vi "cDAQ - UI - Main.vi"() -> ()   [LabVIEW 2011]
uses:
  Controls/Init-Run-End States.ctl
  <vilib>/Utility/miscctls.llb/LVPointTypeDef.ctl
  SubVIs/Controls/TransparencyEffectOperations.ctl
panel:
  in  "Auto Mode":bool
  in  "stop":bool
  out "Picture 2":picture
  out "error out":errorcluster
  out "Picture":picture
  out "Default":picture
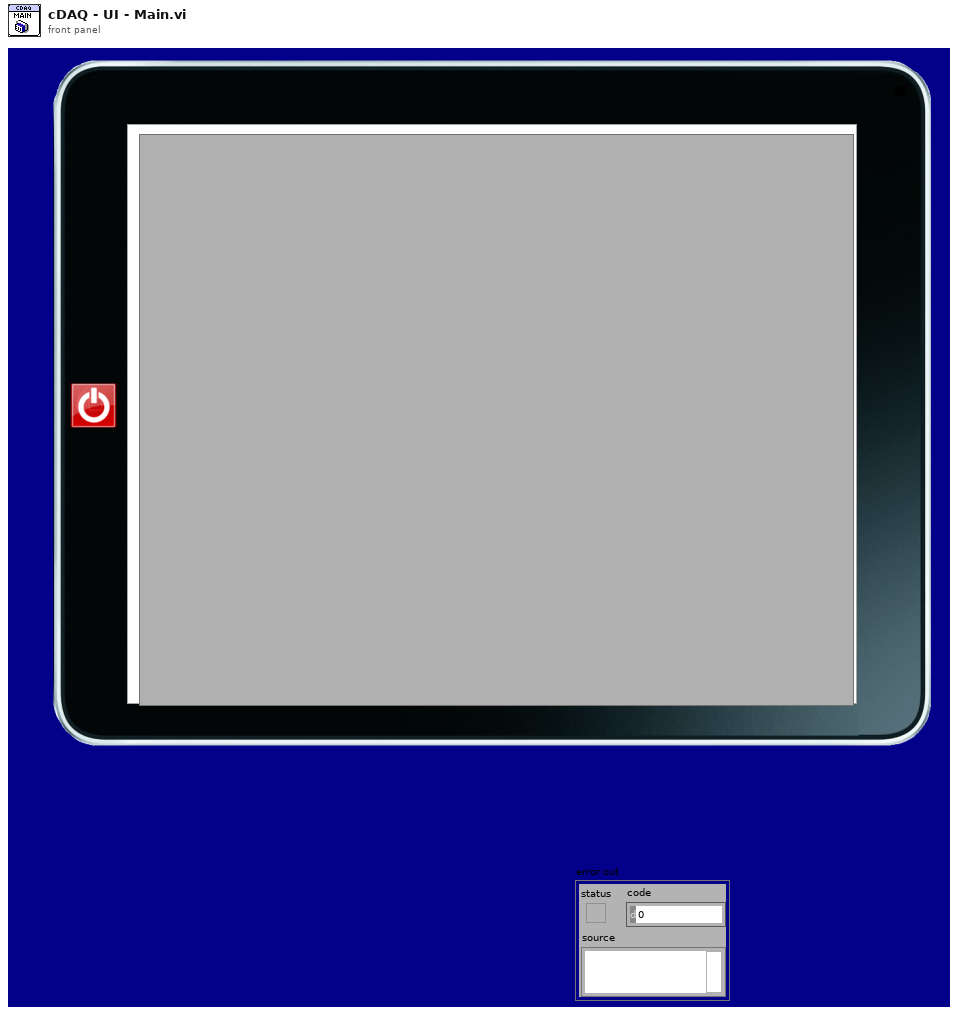
[diagram p1: front panel]
types:
  T1 = typedef "Init-Run-End States.ctl" = enum16{"INIT", "RUN", "END"}
  T2 = typedef "TransparencyEffectOperations.ctl" = enum16{"Show", "Hide 80%", "Hide All"}
  T3 = typedef "LVPointTypeDef.ctl" = cluster{"Horizontal":i16, "Vertical":i16}
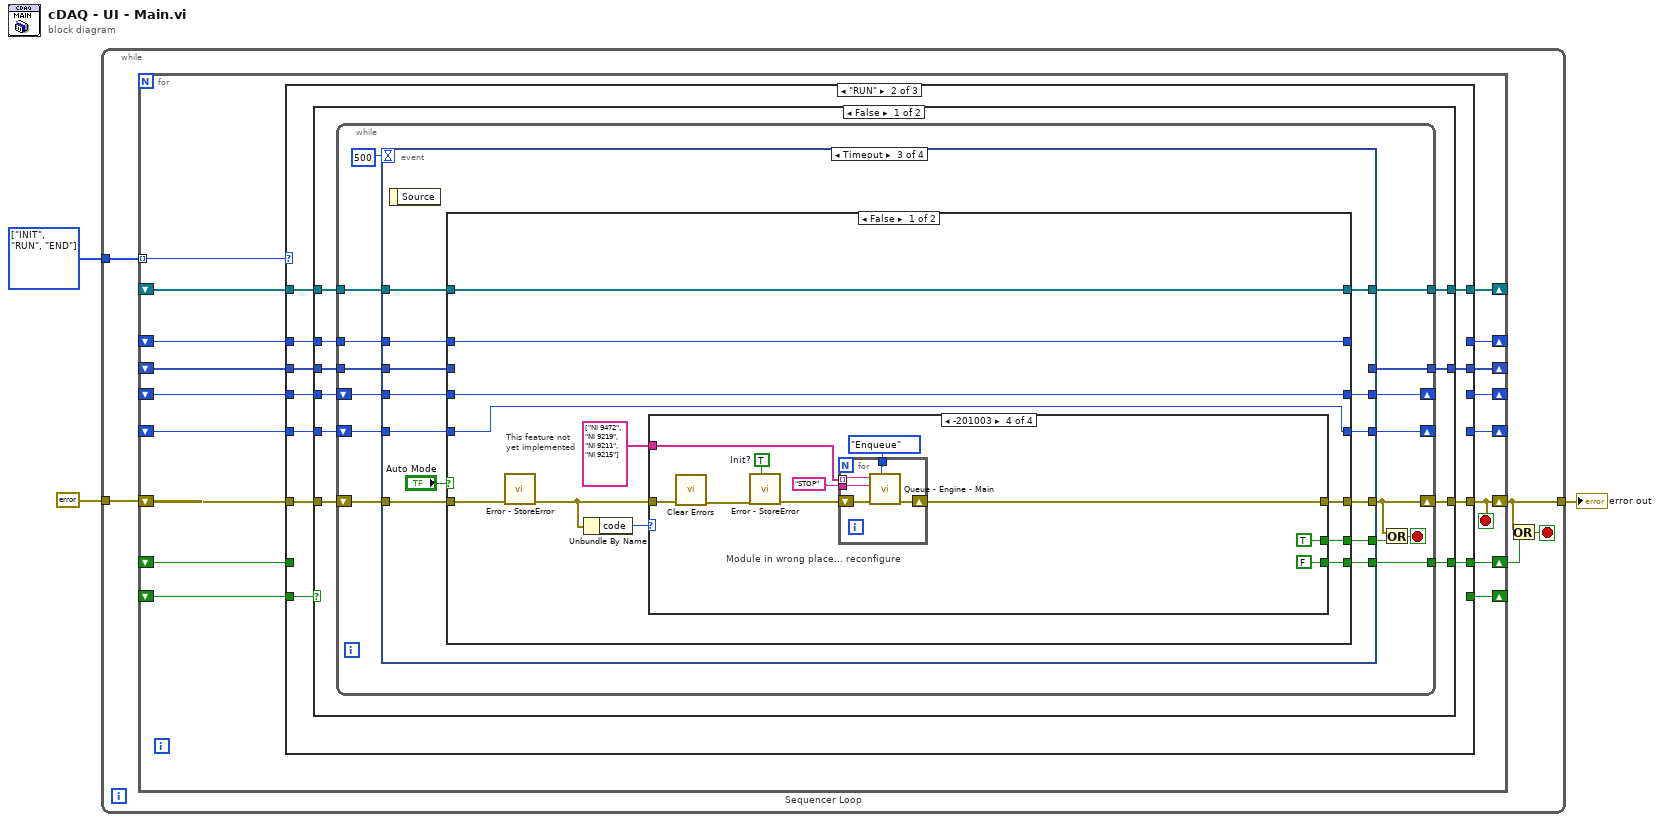
[diagram p0: block diagram]
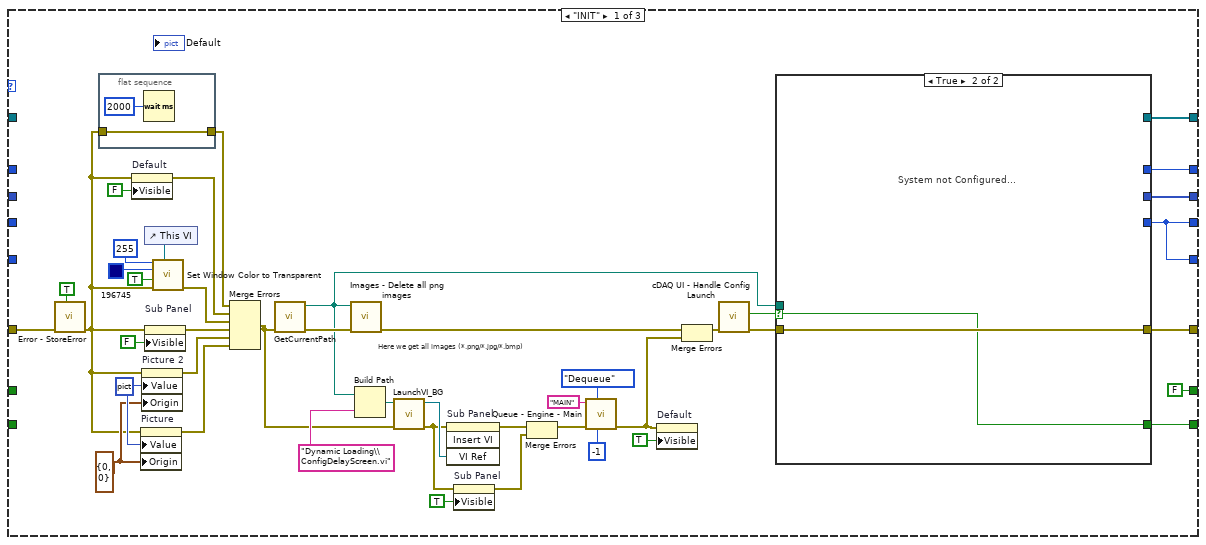
[diagram p2: hidden frame]
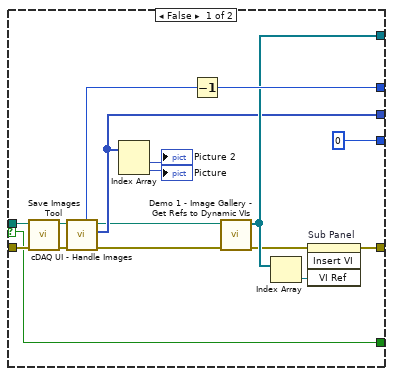
[diagram p3: hidden frame]
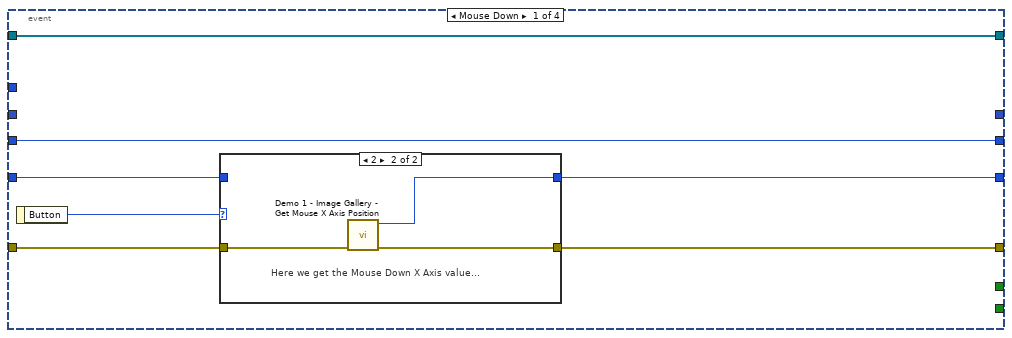
[diagram p4: hidden frame]
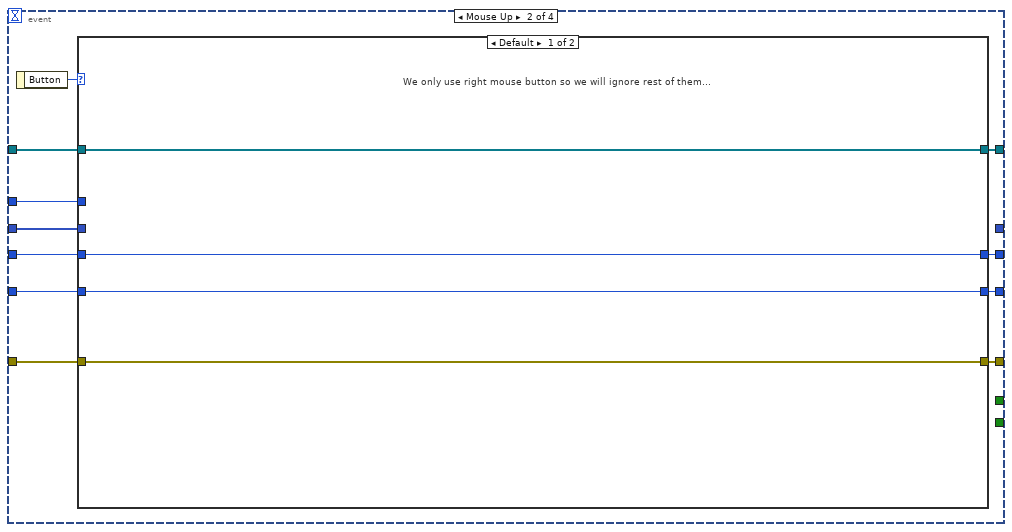
[diagram p6: hidden frame]
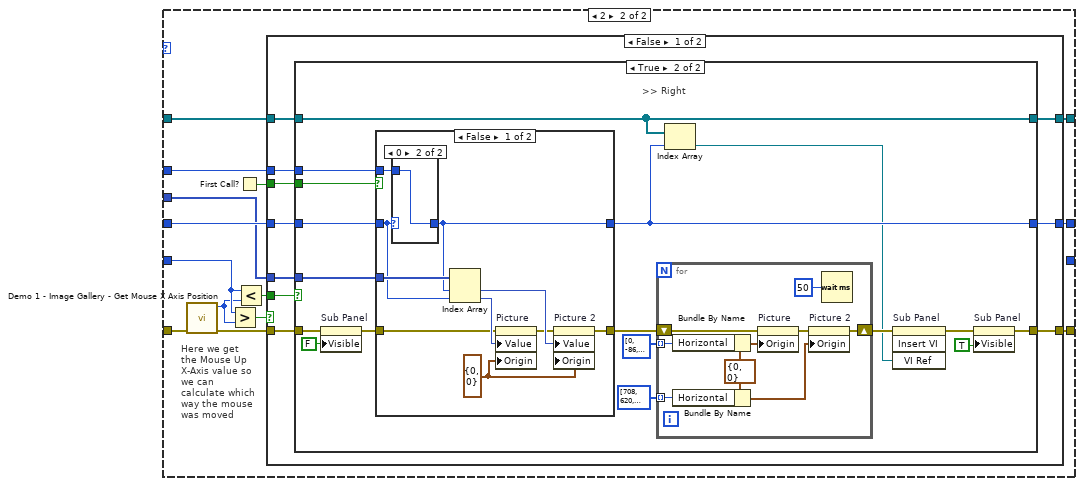
[diagram p7: hidden frame]
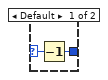
[diagram p9: hidden frame]
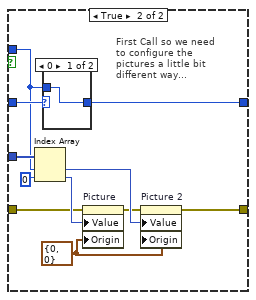
[diagram p10: hidden frame]
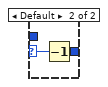
[diagram p11: hidden frame]
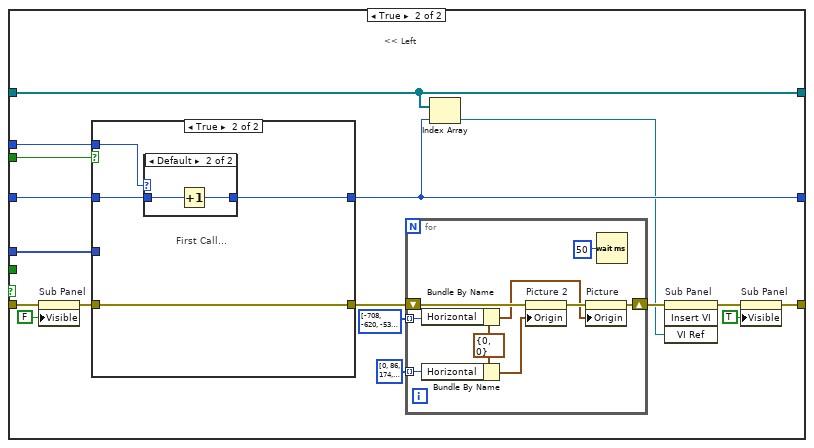
[diagram p12: hidden frame]
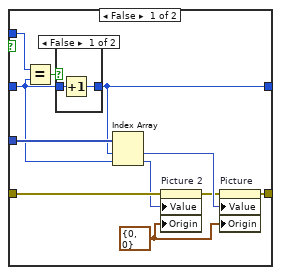
[diagram p13: hidden frame]
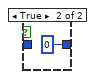
[diagram p14: hidden frame]
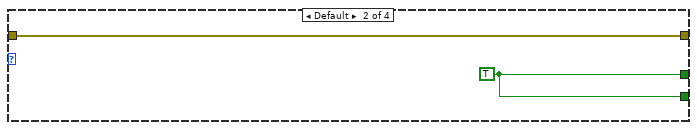
[diagram p17: hidden frame]
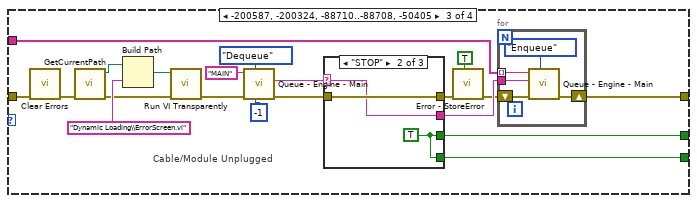
[diagram p18: hidden frame]
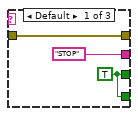
[diagram p19: hidden frame]
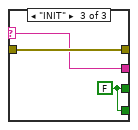
[diagram p20: hidden frame]
diagram:
  w3 = T1[] [enum."INIT", enum."RUN", enum."END"] items=["INIT", "RUN", "END"]
  n1 = while {
    tunnel: w3 -> [w8]
    tunnel: errorcluster {"status"=FALSE, "code"=0, "source"=""} ("error in (no error)") -> [w7]
    tunnel: [w6] -> w1
    stop <- w4 stop-if-true
    n2 = for "Sequencer Loop" {
      tunnel: w8 -> [w20] mode=indexing
      shift-right: [w15] -> w6
      shift-left: w7 -> [w21]
      shift-right: [w19] -> _
      shift-left: _ -> [w22]
      shift-right: [w18] -> _
      shift-left: _ -> [w23]
      shift-right: [w17] -> _
      shift-left: _ -> [w24]
      shift-right: [w16] -> _
      shift-left: _ -> [w25]
      shift-right: [w14] -> _
      shift-left: _ -> [w13]
      shift-right: [w12] -> w5
      shift-left: _ -> [w11]
      shift-right: [w10] -> _
      shift-left: _ -> [w9]
      stop <- w15 stop-if-true
      n3 = case shown="\"RUN\"" w20 {
        tunnel: w25 -> [_ w100 _]
        tunnel: w24 -> [_ w99 _]
        tunnel: w23 -> [_ w98 _]
        tunnel: w22 -> [_ w97 _]
        tunnel: w21 -> [w35 w96 w455]
        tunnel: [w66 w95 w452] -> w15
        tunnel: [w69 _ _] -> w19
        tunnel: [w43 w92 _] -> w18
        tunnel: [w67 _ _] -> w17
        tunnel: [w67 _ _] -> w16
        tunnel: [w65 w93 _] -> w14
        tunnel: w13 -> [_ w94 w454]
        tunnel: [FALSE w91 w451] -> w12
        tunnel: w11 -> [_ _ w451]
        tunnel: [w32 _ _] -> w10
        tunnel: w9 -> [_ w90 _]
        frame "INIT" {
          w52 = picture data[5B] ("Image Out")
          w41 = T3 {"Horizontal"=0, "Vertical"=0} ("Origin")
          # "Here we get all images (*.png/*.jpg/*.bmp)"
          n4 = call "Error - StoreError.vi"("Init?"=TRUE, "Error In"=w35) -> ("Error Out"=w28:errorcluster)  [unwired: 8 in, 1 out]
          n5 = flat-sequence {
            tunnel: w28 -> [w70]
            tunnel: [w70] -> w26
            frame #0 {
              n6 = Wait (ms)(milliseconds to wait=u32 2000) -> ()  [unwired: 1 out]
            }
          }
          n7 = property on="Default" class="Pict"(error in=w28, "Visible"=FALSE) -> (error out=w27:errorcluster)  [unwired: 1 in, 1 out]
          n8 = property on="Picture" class="Pict"(error in=w28, "Value"=w52, "Origin"=w41) -> (error out=w50:errorcluster)  [unwired: 1 in, 1 out]
          n9 = property on="Picture 2" class="Pict"(error in=w28, "Value"=w52, "Origin"=w41) -> (error out=w51:errorcluster)  [unwired: 1 in, 1 out]
          n10 = control-ref of="This VI"() -> (w62:refnum<vi>)
          n11 = property on="Sub Panel" class="SubPnl"(error in=w28, "Visible"=FALSE) -> (error out=w49:errorcluster)  [unwired: 1 in, 1 out]
          n12 = call "Set Window Color to Transparent.vi"("Calling VI's reference"=w62, "error in (no error)"=w28, "Activate"=TRUE, "Color to Replace"=u32 196745, "Factor"=u8 255) -> ("error out"=w45:errorcluster)  [unwired: 3 in]
          n13 = Merge Errors(w26, w27, w45, w49, w51, w50) -> (w40:errorcluster)
          n14 = call "GetCurrentPath.vi"("Error In"=w40) -> ("Error Out"=w38:errorcluster, "Current VI Path Out"=w36:path)  [unwired: 9 in]
          n15 = call "Images - Delete all png images.vi"("Error In"=w38, "Folder In"=w36) -> ("Error Out"=w37:errorcluster)  [unwired: 9 in]
          n16 = Build Path(base path=w36, name or relative path="Dynamic Loading\\ConfigDelayScreen.vi") -> (appended path=w60:path)
          n17 = call "LaunchVI_BG.vi"("error in"=w40, "vi path"=w60) -> ("error out"=w54:errorcluster, "reference out"=w59:refnum<vi>)  [unwired: 8 in]
          n18 = invoke on="Sub Panel" class="SubPanel" method="Insert VI"(error in=w54, "VI Ref"=w59) -> (error out=w47:errorcluster)  [unwired: 2 in, 3 out]
          n19 = property on="Sub Panel" class="SubPnl"(error in=w54, "Visible"=TRUE) -> (error out=w48:errorcluster)  [unwired: 1 in, 1 out]
          n20 = Merge Errors(w47, w48) -> (w46:errorcluster)
          n21 = call "Queue - Engine - Main.vi"("timeout in ms (-1)"=-1, "Operation"=enum16{"Enqueue", "Dequeue", "Flush", "Release"}."Dequeue", "error in"=w46, "Queue Name In"="MAIN") -> ("error out"=w30:errorcluster)  [unwired: 5 in, 2 out]
          n22 = property on="Default" class="Pict"(error in=w30, "Visible"=TRUE) -> ()  [unwired: 1 in, 2 out]
          n23 = Merge Errors(w37, w30) -> (w42:errorcluster)
          n24 = call "cDAQ UI - Handle Config Launch.vi"("error in (no error)"=w42) -> ("error out"=w39:errorcluster, "Not configured?"=w33:bool)  [unwired: 9 in]
          n25 = case shown="True" w33 {
            selector: w33 -> [w72 w88]
            tunnel: [w87 _] -> w69
            tunnel: [0 ("Horizontal") _] -> w67
            tunnel: [w85 w89] -> w66
            tunnel: [w84 _] -> w65
            tunnel: [w78 _] -> w43
            tunnel: w39 -> [w75 w89]
            tunnel: w36 -> [w73 _]
            tunnel: [w72 w88] -> w32
            frame False {
              n26 = call "Save Images Tool.vi"("Error In"=w75) -> ("Error Out"=w74:errorcluster)  [unwired: 10 in]
              n27 = call "cDAQ UI - Handle Images.vi"("error in"=w74, "Current VI Path Out"=w73) -> ("error out"=w76:errorcluster, "Images Out"=w78:picture[], "Dup Path Out"=w77:path, "Nr of Images Out"=w79:i32)  [unwired: 6 in]
              n28 = Index Array(array=w78) -> (element #1=→"Picture 2":picture, element #2=→"Picture":picture)  [unwired: 2 in]
              n29 = Decrement(x=w79) -> (x-1=w87:i32)
              n30 = call "Demo 1 - Image Gallery - Get Refs to Dynamic VIs.vi"("Error In"=w76, "Root Path In"=w77) -> ("Error Out"=w80:errorcluster, "Array"=w84:refnum<vi>[])  [unwired: 8 in]
              n31 = Index Array(array=w84) -> (element=w83:refnum<vi>)  [unwired: 1 in]
              n32 = invoke on="Sub Panel" class="SubPanel" method="Insert VI"(error in=w80, "VI Ref"=w83) -> (error out=w85:errorcluster)  [unwired: 2 in, 3 out]
            }
            frame True {
              # "System not Configured..."
            }
          }
        }
        frame "RUN" {
          n33 = case shown="False" w90 {
            tunnel: w100 -> [w110 _]
            tunnel: w99 -> [w109 _]
            tunnel: w98 -> [w108 _]
            tunnel: w97 -> [w107 _]
            tunnel: w96 -> [w106 w438]
            tunnel: [w105 w437] -> w95
            tunnel: w94 -> [w104 w435]
            tunnel: [w103 w435] -> w93
            tunnel: [w102 _] -> w92
            tunnel: [w101 w436] -> w91
            frame False {
              n34 = while {
                shift-right: [w125] -> _
                shift-left: w110 -> [w124]
                shift-right: [w116] -> w105
                shift-left: w106 -> [w123]
                shift-right: [w119] -> _
                shift-left: w109 -> [w121]
                tunnel: w108 -> [w122]
                tunnel: w104 -> [w115]
                tunnel: [w114] -> w103
                tunnel: [w113] -> w102
                tunnel: [w112] -> w101
                tunnel: w107 -> [w120]
                stop <- w117 stop-if-true
                n35 = event shown="[2] Timeout" {
                  selector: _ -> [_ _ _ _]
                  dyn-events: _ -> [_ _ _ _]
                  timeout: 500 -> [_ _ _ _]
                  tunnel: [_ _ w282 w423] -> w118
                  tunnel: [w129 w139 w280 w424] -> w125
                  tunnel: w124 -> [w127 w148 w292 w424]
                  tunnel: w123 -> [w130 w141 w286 w428]
                  tunnel: [w131 w147 w291 w429] -> w116
                  tunnel: w122 -> [_ w145 w289 w426]
                  tunnel: w121 -> [w132 w146 w290 w425]
                  tunnel: w120 -> [_ w144 w288 _]
                  tunnel: [w132 w143 w287 w425] -> w119
                  tunnel: w115 -> [w126 w142 w285 w431]
                  tunnel: [w126 w138 w284 w431] -> w114
                  tunnel: [_ _ _ w426] -> w113
                  tunnel: [_ _ w281 w422] -> w112
                  event Mouse Down {
                    n36 = event-data() -> ("Button"=w128:u16)  [unwired: 1 in]
                    n37 = case shown="2" w128 {
                      tunnel: [w133 w137] -> w131
                      tunnel: w130 -> [w133 w136]
                      tunnel: [w134 w135] -> w129
                      tunnel: w127 -> [w134 _]
                      frame Default {
                      }
                      frame 2 {
                        # "Here we get the Mouse Down X Axis value..."
                        n38 = call "Demo 1 - Image Gallery - Get Mouse X Axis Position.vi"("Error In"=w136) -> ("Error Out"=w137:errorcluster, "Mouse X Axis Out"=w135:i32)  [unwired: 9 in]
                      }
                    }
                  }
                  event Mouse Up {
                    n39 = event-data() -> ("Button"=w140:u16)  [unwired: 1 in]
                    n40 = case shown="Default" w140 {
                      tunnel: w148 -> [w150 w166]
                      tunnel: [w152 w163] -> w147
                      tunnel: w146 -> [w151 w162]
                      tunnel: w145 -> [_ w161]
                      tunnel: w144 -> [_ w160]
                      tunnel: [w151 w159] -> w143
                      tunnel: w142 -> [w149 w155]
                      tunnel: w141 -> [w152 w154]
                      tunnel: [w150 _] -> w139
                      tunnel: [w149 w153] -> w138
                      frame Default {
                        # "We only use right mouse button so we will ignore rest of them..."
                      }
                      frame 2 {
                        # "Here we get the Mouse Up X-Axis value so we can calculate which way the mouse was moved"
                        n41 = call "Demo 1 - Image Gallery - Get Mouse X Axis Position.vi"("Error In"=w154) -> ("Error Out"=w157:errorcluster, "Mouse X Axis Out"=w156:i32)  [unwired: 9 in]
                        n42 = Greater?(x=w166, y=w156) -> (0:w164:bool)
                        n43 = First Call?() -> (First Call?: T/F=w158:bool)
                        n44 = Less?(x=w166, y=w156) -> (x < y?=w165:bool)
                        n45 = case shown="False" w164 {
                          tunnel: w165 -> [w176 _]
                          tunnel: w157 -> [w175 w237]
                          tunnel: [w174 w240] -> w163
                          tunnel: w162 -> [w173 w249]
                          tunnel: w161 -> [w172 w246]
                          tunnel: w160 -> [w171 w248]
                          tunnel: [w170 w235] -> w159
                          tunnel: w158 -> [w169 w245]
                          tunnel: w155 -> [w168 w233]
                          tunnel: [w167 w233] -> w153
                          frame False {
                            n46 = case shown="True" w176 {
                              tunnel: w175 -> [w179 w184]
                              tunnel: [w179 w185] -> w174
                              tunnel: w173 -> [w178 w194]
                              tunnel: w172 -> [_ w195]
                              tunnel: w171 -> [_ w196]
                              tunnel: [w178 w189] -> w170
                              tunnel: w169 -> [_ w192]
                              tunnel: w168 -> [w177 w180]
                              tunnel: [w177 w180] -> w167
                              frame False {
                                # "No movement"
                              }
                              frame True {
                                # ">> Right"
                                n47 = property on="Sub Panel" class="SubPnl"(error in=w184, "Visible"=FALSE) -> (error out=w183:errorcluster)  [unwired: 1 in, 1 out]
                                n48 = case shown="False" w192 {
                                tunnel: w196 -> [w206 w210]
                                tunnel: w195 -> [w205 w219]
                                tunnel: [w198 w212] -> w189
                                tunnel: w194 -> [w197 w211]
                                tunnel: w183 -> [w199 w214]
                                tunnel: [w201 w213] -> w193
                                frame False {
                                w203 = T3 {"Horizontal"=0, "Vertical"=0} ("Origin")
                                n49 = case shown="0" w197 {
                                selector: w197 -> [w207 _]
                                tunnel: [w208 w209] -> w198
                                tunnel: w206 -> [_ w209]
                                frame Default {
                                n50 = Decrement(x=w207) -> (x-1=w208:i32)
                                }
                                frame 0 {
                                }
                                }
                                n51 = Index Array(array=w205, index #1=w198, index #2=w197) -> (element #1=w204:picture, element #2=w200:picture)
                                n52 = property on="Picture" class="Pict"(error in=w199, "Value"=w200, "Origin"=w203) -> (error out=w202:errorcluster)  [unwired: 1 in, 1 out]
                                n53 = property on="Picture 2" class="Pict"(error in=w202, "Value"=w204, "Origin"=w203) -> (error out=w201:errorcluster)  [unwired: 1 in, 1 out]
                                }
                                frame True {
                                w220 = T3 {"Horizontal"=0, "Vertical"=0} ("Origin")
                                # "First Call so we need to configure the pictures a little bit different way..."
                                n54 = Index Array(array=w219, index #1=w210, index #2=0 ("index")) -> (element #1=w217:picture, element #2=w216:picture)
                                n55 = case shown="0" w211 {
                                selector: w211 -> [_ w222]
                                tunnel: [w221 w223] -> w212
                                tunnel: w210 -> [w221 _]
                                frame 0 {
                                }
                                frame Default {
                                n56 = Decrement(x=w222) -> (x-1=w223:i32)
                                }
                                }
                                n57 = property on="Picture" class="Pict"(error in=w214, "Value"=w216, "Origin"=w220) -> (error out=w215:errorcluster)  [unwired: 1 in, 1 out]
                                n58 = property on="Picture 2" class="Pict"(error in=w215, "Value"=w217, "Origin"=w220) -> (error out=w213:errorcluster)  [unwired: 1 in, 1 out]
                                }
                                }
                                n59 = for {
                                tunnel: i16[] [708, 620, 530, 440, 354, 264, 174, 86, 0] ("Array") -> [w227] mode=indexing
                                shift-right: [w225] -> w188
                                shift-left: w193 -> [w229]
                                tunnel: i16[] [0, -86, -174, -264, -354, -440, -530, -620, -708] ("reversed array") -> [w224] mode=indexing
                                w231 = T3 {"Horizontal"=0, "Vertical"=0} ("Origin")
                                n60 = Bundle By Name(cluster=w231, "Horizontal"=w224) -> (w230:T3)
                                n61 = Bundle By Name(cluster=w231, "Horizontal"=w227) -> (w232:T3)
                                n62 = property on="Picture" class="Pict"(error in=w229, "Origin"=w230) -> (error out=w226:errorcluster)  [unwired: 1 in, 1 out]
                                n63 = property on="Picture 2" class="Pict"(error in=w226, "Origin"=w232) -> (error out=w225:errorcluster)  [unwired: 1 in, 1 out]
                                n64 = Wait (ms)(milliseconds to wait=u32 50) -> ()  [unwired: 1 out]
                                }
                                n65 = Index Array(array=w180, index=w189) -> (element=w181:refnum<vi>)
                                n66 = invoke on="Sub Panel" class="SubPanel" method="Insert VI"(error in=w188, "VI Ref"=w181) -> (error out=w187:errorcluster)  [unwired: 2 in, 3 out]
                                n67 = property on="Sub Panel" class="SubPnl"(error in=w187, "Visible"=TRUE) -> (error out=w185:errorcluster)  [unwired: 1 in, 1 out]
                              }
                            }
                          }
                          frame True {
                            # "<< Left"
                            n68 = property on="Sub Panel" class="SubPnl"(error in=w237, "Visible"=FALSE) -> (error out=w238:errorcluster)  [unwired: 1 in, 1 out]
                            n69 = case shown="True" w245 {
                              tunnel: w249 -> [w252 w267]
                              tunnel: w248 -> [w250 w264]
                              tunnel: [w259 w266] -> w247
                              tunnel: w246 -> [w258 _]
                              tunnel: [w257 w265] -> w235
                              tunnel: w238 -> [w253 w266]
                              frame False {
                                w256 = T3 {"Horizontal"=0, "Vertical"=0} ("Origin")
                                n70 = Equal?(x=w250, y=w252) -> (x = y?=w260:bool)
                                n71 = case shown="False" w260 {
                                tunnel: [w261 0] -> w257
                                tunnel: w252 -> [w262 _]
                                frame False {
                                n72 = Increment(x=w262) -> (x+1=w261:i32)
                                }
                                frame True {
                                }
                                }
                                n73 = Index Array(array=w258, index #1=w257, index #2=w252) -> (element #1=w255:picture, element #2=w251:picture)
                                n74 = property on="Picture 2" class="Pict"(error in=w253, "Value"=w251, "Origin"=w256) -> (error out=w254:errorcluster)  [unwired: 1 in, 1 out]
                                n75 = property on="Picture" class="Pict"(error in=w254, "Value"=w255, "Origin"=w256) -> (error out=w259:errorcluster)  [unwired: 1 in, 1 out]
                              }
                              frame True {
                                # "First Call..."
                                n76 = case shown="Default" w264 {
                                selector: w264 -> [w268 _]
                                tunnel: w267 -> [_ w270]
                                tunnel: [w268 w269] -> w265
                                frame 0 {
                                }
                                frame Default {
                                n77 = Increment(x=w270) -> (x+1=w269:i32)
                                }
                                }
                              }
                            }
                            n78 = for {
                              tunnel: i16[] [0, 86, 174, 264, 352, 440, 530, 620, 708] ("reversed array") -> [w277] mode=indexing
                              shift-right: [w273] -> w242
                              shift-left: w247 -> [w275]
                              tunnel: i16[] [-708, -620, -530, -440, -352, -264, -174, -86, 0] ("reversed array 2") -> [w271] mode=indexing
                              w278 = T3 {"Horizontal"=0, "Vertical"=0} ("Origin")
                              n79 = Bundle By Name(cluster=w278, "Horizontal"=w271) -> (w272:T3)
                              n80 = Bundle By Name(cluster=w278, "Horizontal"=w277) -> (w279:T3)
                              n81 = property on="Picture 2" class="Pict"(error in=w275, "Origin"=w279) -> (error out=w274:errorcluster)  [unwired: 1 in, 1 out]
                              n82 = property on="Picture" class="Pict"(error in=w274, "Origin"=w272) -> (error out=w273:errorcluster)  [unwired: 1 in, 1 out]
                              n83 = Wait (ms)(milliseconds to wait=u32 50) -> ()  [unwired: 1 out]
                            }
                            n84 = Index Array(array=w233, index=w235) -> (element=w234:refnum<vi>)
                            n85 = invoke on="Sub Panel" class="SubPanel" method="Insert VI"(error in=w242, "VI Ref"=w234) -> (error out=w241:errorcluster)  [unwired: 2 in, 3 out]
                            n86 = property on="Sub Panel" class="SubPnl"(error in=w241, "Visible"=TRUE) -> (error out=w240:errorcluster)  [unwired: 1 in, 1 out]
                          }
                        }
                      }
                    }
                  }
                  event Timeout {
                    n87 = event-data() -> ()  [unwired: 1 in, 1 out]
                    n88 = case shown="False" "Auto Mode" {
                      tunnel: w292 -> [w294 _]
                      tunnel: [w297 w374] -> w291
                      tunnel: w290 -> [w302 w373]
                      tunnel: w289 -> [_ w372]
                      tunnel: w288 -> [w301 w371]
                      tunnel: [w302 w370] -> w287
                      tunnel: w286 -> [w300 w358]
                      tunnel: w285 -> [w303 w359]
                      tunnel: [w303 w359] -> w284
                      tunnel: [w301 w357] -> _
                      tunnel: [w296 _] -> w282
                      tunnel: [w295 _] -> w281
                      tunnel: [w294 _] -> w280
                      frame False {
                        # "This feature not yet implemented"
                        n89 = call "Error - StoreError.vi"("Error In"=w300) -> ("Error Out"=w298:errorcluster)  [unwired: 9 in, 1 out]
                        n90 = Unbundle By Name(w298) -> ("code"=w299:i32)
                        n91 = case shown="-201003" w299 {
                          tunnel: w298 -> [w304 w306 w314 w344]
                          tunnel: [w304 w306 w312 w348] -> w297
                          tunnel: [_ w305 w317 TRUE] -> w296
                          tunnel: [_ w305 w316 FALSE] -> w295
                          tunnel: string[] ["NI 9472", "NI 9219", "NI 9211", "NI 9215"] ("Error Sources Out") -> [_ _ w307 w347]
                          frame 0 {
                          }
                          frame Default {
                            w305 = TRUE
                          }
                          frame -200587, -200324, -88710..-88708, -50405 {
                            # "Cable/Module Unplugged"
                            n92 = call <vilib>:"Clear Errors.vi"("error in (no error)"=w314) -> ("error out"=w315:errorcluster)  [unwired: 6 in]
                            n93 = call "GetCurrentPath.vi"("Error In"=w315) -> ("Error Out"=w324:errorcluster, "Current VI Path Out"=w325:path)  [unwired: 9 in]
                            n94 = Build Path(base path=w325, name or relative path="Dynamic Loading\\ErrorScreen.vi") -> (appended path=w322:path)
                            n95 = call "Run VI Transparently.vi"("error in"=w324, "vi path"=w322) -> ("error out"=w323:errorcluster)  [unwired: 9 in]
                            n96 = call "Queue - Engine - Main.vi"("timeout in ms (-1)"=-1, "Operation"=enum16{"Enqueue", "Dequeue", "Flush", "Release"}."Dequeue", "error in"=w323, "Queue Name In"="MAIN") -> ("error out"=w313:errorcluster, "Data Out"=w318:string)  [unwired: 5 in, 1 out]
                            n97 = case shown="\"STOP\"" w318 {
                              selector: w318 -> [_ w335 w339]
                              tunnel: [w334 w337 w338] -> w317
                              tunnel: [w334 w337 w338] -> w316
                              tunnel: w313 -> [w333 w336 w340]
                              tunnel: [w333 w336 w340] -> w309
                              tunnel: ["STOP" ("name or relative path") w335 w339] -> w311
                              frame Default {
                                w334 = TRUE
                              }
                              frame "STOP" {
                                w337 = TRUE
                              }
                              frame "INIT" {
                                w338 = FALSE
                              }
                            }
                            n98 = call "Error - StoreError.vi"("Init?"=TRUE, "Error In"=w309) -> ("Error Out"=w308:errorcluster)  [unwired: 8 in, 1 out]
                            n99 = for {
                              tunnel: w311 -> [w329]
                              tunnel: w307 -> [w327] mode=indexing
                              shift-right: [w331] -> w312
                              shift-left: w308 -> [w328]
                              n100 = call "Queue - Engine - Main.vi"("Operation"=enum16{"Enqueue", "Dequeue", "Flush", "Release"}."Enqueue", "error in"=w328, "Queue Data In"=w329, "Queue Name In"=w327) -> ("error out"=w331:errorcluster)  [unwired: 5 in, 2 out]
                            }
                          }
                          frame -201003 {
                            w350 = TRUE  # Init?
                            # "Module in wrong place... reconfigure"
                            n101 = call <vilib>:"Clear Errors.vi"("error in (no error)"=w344) -> ("error out"=w343:errorcluster)  [unwired: 6 in]
                            n102 = call "Error - StoreError.vi"("Init?"=w350, "Error In"=w343) -> ("Error Out"=w349:errorcluster)  [unwired: 8 in, 1 out]
                            n103 = for {
                              tunnel: "STOP" ("name or relative path") -> [w354]
                              tunnel: w347 -> [w352] mode=indexing
                              shift-right: [w355] -> w348
                              shift-left: w349 -> [w353]
                              tunnel: enum16{"Enqueue", "Dequeue", "Flush", "Release"}."Enqueue" ("Operation") -> [w351]
                              n104 = call "Queue - Engine - Main.vi"("Operation"=w351, "error in"=w353, "Queue Data In"=w354, "Queue Name In"=w352) -> ("error out"=w355:errorcluster)  [unwired: 5 in, 2 out]
                            }
                          }
                        }
                      }
                      frame True {
                        # ">> Right"
                        n105 = Wait (ms)(milliseconds to wait=u32 5000) -> ()  [unwired: 1 out]
                        n106 = property on="Sub Panel" class="SubPnl"(error in=w358, "Visible"=FALSE) -> (error out=w362:errorcluster)  [unwired: 1 in, 1 out]
                        n107 = First Call?() -> (First Call?: T/F=w369:bool)
                        n108 = case shown="False" w369 {
                          tunnel: w371 -> [w385 w396]
                          tunnel: w372 -> [w384 w398]
                          tunnel: [w378 w401] -> w370
                          tunnel: w373 -> [w376 w400]
                          tunnel: w362 -> [w377 w392]
                          tunnel: [w380 w391] -> w368
                          tunnel: [w375 w390] -> w357
                          frame False {
                            w382 = T3 {"Horizontal"=0, "Vertical"=0} ("Origin")
                            n109 = case shown="0" w376 {
                              selector: w376 -> [w387 _]
                              tunnel: [w388 w389] -> w378
                              tunnel: w385 -> [w386 w389]
                              tunnel: [w386 w389] -> w375
                              frame Default {
                                n110 = Decrement(x=w387) -> (x-1=w388:i32)
                              }
                              frame 0 {
                              }
                            }
                            n111 = Index Array(array=w384, index #1=w378, index #2=w376) -> (element #1=w383:picture, element #2=w379:picture)
                            n112 = property on="Picture" class="Pict"(error in=w377, "Value"=w379, "Origin"=w382) -> (error out=w381:errorcluster)  [unwired: 1 in, 1 out]
                            n113 = property on="Picture 2" class="Pict"(error in=w381, "Value"=w383, "Origin"=w382) -> (error out=w380:errorcluster)  [unwired: 1 in, 1 out]
                          }
                          frame True {
                            w399 = T3 {"Horizontal"=0, "Vertical"=0} ("Origin")
                            # "First Call so we need to configure the pictures a little bit different way..."
                            n114 = Index Array(array=w398, index #1=w396, index #2=0 ("index")) -> (element #1=w395:picture, element #2=w394:picture)
                            n115 = case shown="0" w400 {
                              selector: w400 -> [_ w404]
                              tunnel: [w402 w405] -> w401
                              tunnel: w396 -> [w402 w403]
                              tunnel: [w402 w403] -> w390
                              frame 0 {
                              }
                              frame Default {
                                n116 = Decrement(x=w404) -> (x-1=w405:i32)
                              }
                            }
                            n117 = property on="Picture" class="Pict"(error in=w392, "Value"=w394, "Origin"=w399) -> (error out=w393:errorcluster)  [unwired: 1 in, 1 out]
                            n118 = property on="Picture 2" class="Pict"(error in=w393, "Value"=w395, "Origin"=w399) -> (error out=w391:errorcluster)  [unwired: 1 in, 1 out]
                          }
                        }
                        n119 = Index Array(array=w359, index=w370) -> (element=w360:refnum<vi>)
                        n120 = for {
                          tunnel: i16[] [708, 620, 530, 440, 354, 264, 174, 86, 0] ("Array") -> [w409] mode=indexing
                          shift-right: [w407] -> w365
                          shift-left: w368 -> [w411]
                          tunnel: i16[] [0, -86, -174, -264, -354, -440, -530, -620, -708] ("reversed array") -> [w406] mode=indexing
                          w413 = T3 {"Horizontal"=0, "Vertical"=0} ("Origin")
                          n121 = Bundle By Name(cluster=w413, "Horizontal"=w406) -> (w412:T3)
                          n122 = Bundle By Name(cluster=w413, "Horizontal"=w409) -> (w414:T3)
                          n123 = property on="Picture" class="Pict"(error in=w411, "Origin"=w412) -> (error out=w408:errorcluster)  [unwired: 1 in, 1 out]
                          n124 = property on="Picture 2" class="Pict"(error in=w408, "Origin"=w414) -> (error out=w407:errorcluster)  [unwired: 1 in, 1 out]
                          n125 = Wait (ms)(milliseconds to wait=u32 50) -> ()  [unwired: 1 out]
                        }
                        n126 = invoke on="Sub Panel" class="SubPanel" method="Insert VI"(error in=w365, "VI Ref"=w360) -> (error out=w364:errorcluster)  [unwired: 2 in, 3 out]
                        n127 = property on="Sub Panel" class="SubPnl"(error in=w364, "Visible"=TRUE) -> (error out=w374:errorcluster)  [unwired: 1 in, 1 out]
                      }
                    }
                  }
                  event "stop": Value Change {
                    n128 = event-data() -> ()  [unwired: 1 in, 1 out]
                    n129 = call "GetCurrentPath.vi"("Error In"=w428) -> ("Error Out"=w421:errorcluster, "Current VI Path Out"=w427:path)  [unwired: 9 in]
                    n130 = Build Path(base path=w427, name or relative path="Dynamic Loading\\StopScreen.vi") -> (appended path=w419:path)
                    n131 = call "Run VI Transparently.vi"("error in"=w421, "vi path"=w419) -> ("error out"=w420:errorcluster)  [unwired: 9 in]
                    n132 = call "Queue - Engine - Main.vi"("timeout in ms (-1)"=-1, "Operation"=enum16{"Enqueue", "Dequeue", "Flush", "Release"}."Dequeue", "error in"=w420, "Queue Name In"="MAIN") -> ("error out"=w429:errorcluster, "Data Out"=w415:string)  [unwired: 5 in, 1 out]
                    n133 = case shown="\"CANCEL\"" w415 {
                      tunnel: [w432 w433 _ TRUE] -> w423
                      tunnel: [w432 w433 _ _] -> w422
                      frame Default {
                        w432 = TRUE
                      }
                      frame "STOP" {
                        w433 = TRUE
                      }
                      frame "CANCEL" {
                      }
                      frame "INIT" {
                      }
                    }
                  }
                }
                n134 = Or(x=w116, y=w118) -> (x .or. y?=w117:bool)
              }
            }
            frame True {
              # "User Selection"
              # "Not configured so we launch \"Not Configured Screen\""
              n135 = call "GetCurrentPath.vi"("Error In"=w438) -> ("Error Out"=w445:errorcluster, "Current VI Path Out"=w446:path)  [unwired: 9 in]
              n136 = Build Path(base path=w446, name or relative path="Dynamic Loading\\NotConfiguredScreen.vi") -> (appended path=w443:path)
              n137 = call "Run VI Transparently.vi"("error in"=w445, "vi path"=w443) -> ("error out"=w444:errorcluster)  [unwired: 9 in]
              n138 = call "Queue - Engine - Main.vi"("timeout in ms (-1)"=-1, "Operation"=enum16{"Enqueue", "Dequeue", "Flush", "Release"}."Dequeue", "error in"=w444, "Queue Name In"="MAIN") -> ("error out"=w437:errorcluster, "Data Out"=w439:string)  [unwired: 5 in, 1 out]
              n139 = case shown="\"INIT\"" w439 {
                tunnel: [TRUE TRUE FALSE] -> w436
                frame Default {
                }
                frame "STOP" {
                }
                frame "INIT" {
                }
              }
            }
          }
        }
        frame "END" {
          n140 = Close Reference(reference=w454, error in (no error)=w455) -> (error out=w453:errorcluster)
          n141 = case shown="False" w451 {
            tunnel: w453 -> [w456 w461]
            tunnel: [w456 w458] -> w452
            frame False {
            }
            frame True {
              n142 = control-ref of="This VI"() -> (w457:refnum<vi>)
              n143 = call "TransparencyEffect.vi"("Operation"=TransparencyEffectOperations."Hide All", "error in"=w461, "VI Ref in"=w457) -> ("error out"=w459:errorcluster)  [unwired: 8 in]
              n144 = invoke class="VI" method="FP.Close"(reference=w457, error in=w459) -> (error out=w458:errorcluster)  [unwired: 1 in, 2 out]
            }
          }
        }
      }
    }
    n145 = Or(x=w6, y=w5) -> (x .or. y?=w4:bool)
  }
  "error out" <- w1
